vi "UpdateCallerDisplay.vi"(8 "error in (no error)":errorcluster, 10 "Message":string, 11 "Caller in":refnum<class "Caller.lvclass">) -> (0 "error out":errorcluster, 3 "Caller out":refnum<class "Caller.lvclass">)   [LabVIEW 2020, in "Caller.lvlib" / "Caller.lvclass"]
uses:
  Caller.lvclass
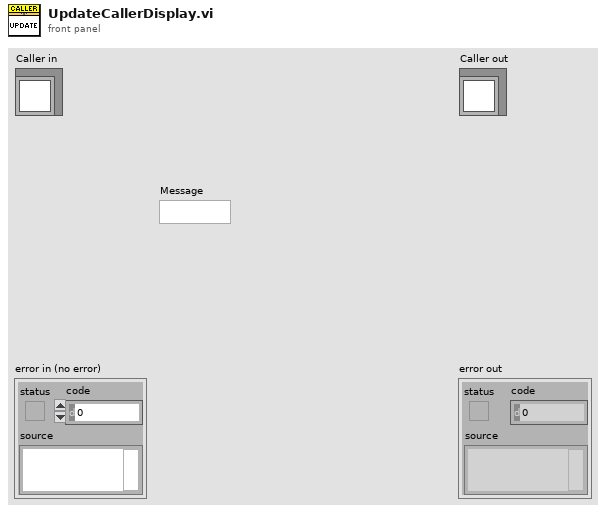
[diagram p1: front panel]
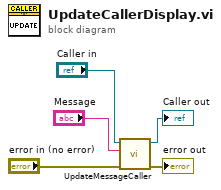
[diagram p0: block diagram]
diagram:
  n1 = call "UpdateMessageCaller.vi"("error in (no error)"="error in (no error)", "Message"="Message", "Caller in"="Caller in") -> ("error out"=→"error out":errorcluster, "Caller out"=→"Caller out":refnum<class "Caller.lvclass">)  [unwired: 7 in]
